vi "To String Array.vi"(8 "error in (no error)":errorcluster, 11 "Update Tag Config in":refnum<class "Update Tag Config.lvclass">) -> (0 "error out":errorcluster, 1 "Step String Array":string[](array[string]), 3 "Update Tag Config out":refnum<class "Update Tag Config.lvclass">)   [LabVIEW 2015, in "Update Tag Config.lvclass"]
uses:
  Update Tag Config.lvclass
  <vilib>/NI/Tag Bus/tag/tag descriptor.lvclass/tag descriptor.ctl
  <vilib>/NI/Tag Bus Module Framework/channel/TBM channel.lvclass
  classes/Step/Config/Step Config.lvclass
  <vilib>/NI/Tag Bus/tag/tag descriptor.lvclass
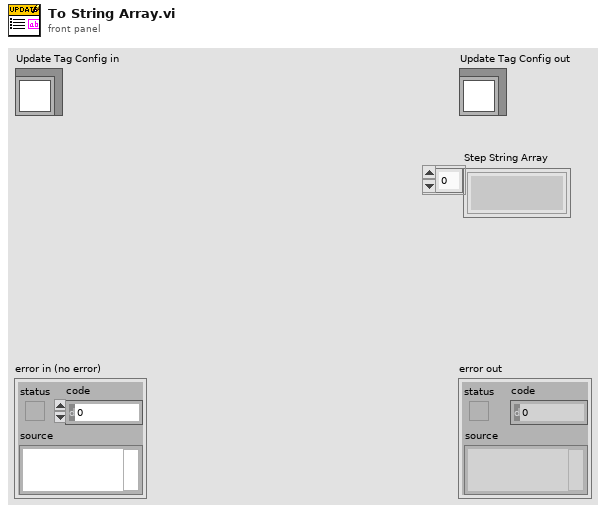
[diagram p1: front panel]
types:
  T1 = typedef "tag bus.lvlib/tag descriptor.lvclass/Data Type.ctl" = enum16{"Double", "Single", "I64", "I32", "I16", "I8", "U64", "U32", "U16", "U8", "Boolean", "String", "Array of Double", "Array of Single", "Array of I64", "Array of I32", "Array of I16", "Array of I8", "Array of U64", "Array of U32", "Array of U16", "Array of U8", "Array of Boolean", "Array of String"}
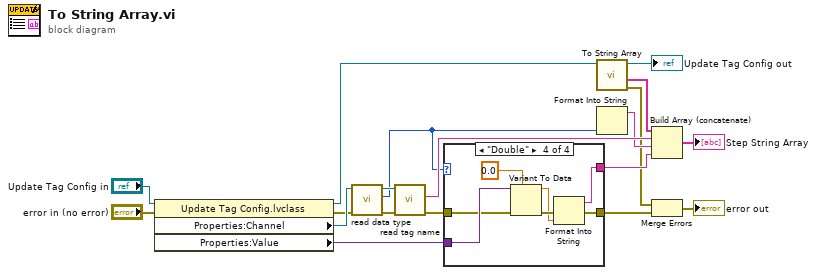
[diagram p0: block diagram]
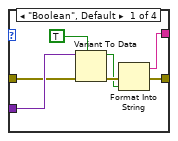
[diagram p2: hidden frame]
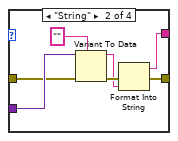
[diagram p3: hidden frame]
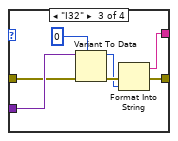
[diagram p4: hidden frame]
diagram:
  n1 = property class="Update Tag Config.lvclass"(reference="Update Tag Config in", error in="error in (no error)") -> (reference out=w6:refnum<class "Update Tag Config.lvclass">, error out=w9:errorcluster, "Properties:Channel"=w16:refnum<class "TBM channel.lvclass">, "Properties:Value"=w12:variant)
  n2 = call <vilib>:"read data type.vi"("error in"=w9, "system tag in"=w16) -> ("error out"=w8:errorcluster, "data type"=w11:T1, "system tag out"=w17:refnum<class "TBM channel.lvclass">)  [unwired: 7 in]
  n3 = call <vilib>:"read tag name.vi"("error in"=w8, "system tag in"=w17) -> ("error out"=w7:errorcluster, "name"=w15:string)  [unwired: 7 in, 1 out]
  n4 = case shown="\"Double\"" w11 {
    tunnel: w12 -> [w26 w33 w40 w47]
    tunnel: [w22 w29 w36 w43] -> w10
    tunnel: [w21 w28 w35 w42] -> w3
    tunnel: w7 -> [w20 w27 w34 w41]
    frame "Boolean", Default {
      n5 = Variant To Data(error in=w20, type=TRUE, Variant=w26) -> (data=w23:bool, error out=w24:errorcluster)
      n6 = Format Into String(error in=w24, w23) -> (resulting string=w22:string, error out=w21:errorcluster)  [unwired: 2 in]
    }
    frame "String" {
      n7 = Variant To Data(error in=w27, type="", Variant=w33) -> (data=w30:string, error out=w31:errorcluster)
      n8 = Format Into String(error in=w31, w30) -> (resulting string=w29:string, error out=w28:errorcluster)  [unwired: 2 in]
    }
    frame "I32" {
      n9 = Variant To Data(error in=w34, type=0, Variant=w40) -> (data=w37:i32, error out=w38:errorcluster)
      n10 = Format Into String(error in=w38, w37) -> (resulting string=w36:string, error out=w35:errorcluster)  [unwired: 2 in]
    }
    frame "Double" {
      n11 = Variant To Data(error in=w41, type=0.0, Variant=w47) -> (data=w44:dbl, error out=w45:errorcluster)
      n12 = Format Into String(error in=w45, w44) -> (resulting string=w43:string, error out=w42:errorcluster)  [unwired: 2 in]
    }
  }
  n13 = call-parent "To String Array.vi"("Step Config in"=w6) -> ("error out"=w2:errorcluster, "Step String Array"=w4:string[], "Step Config out"=→"Update Tag Config out":refnum<class "Update Tag Config.lvclass">)  [unwired: 8 in]
  n14 = Format Into String(w11) -> (resulting string=w13:string)  [unwired: 3 in, 1 out]
  n15 = Build Array (concatenate)(w4, w15, w13, w10) -> (→"Step String Array":string[])
  n16 = Merge Errors(w2, w3) -> (→"error out":errorcluster)
